vi "Pose3d_Log_Orig.vi"(9 "end Pose3d":T2={"Translation3d"={"X"=0.0, "Y"=0.0, "Z"=0.0}, "Rotation3d"={"Q_quaternion"={"R"=1.0, "V"=[0.0, 0.0, 0.0]}}} {"Translation3d"."Z" format="%14.3f"; "Translation3d"."Y" format="%14.3f"; "Translation3d"."X" format="%14.3f"}, 11 "in Pose3d":T2={"Translation3d"={"X"=0.0, "Y"=0.0, "Z"=0.0}, "Rotation3d"={"Q_quaternion"={"R"=1.0, "V"=[0.0, 0.0, 0.0]}}} {"Translation3d"."Z" format="%14.3f"; "Translation3d"."Y" format="%14.3f"; "Translation3d"."X" format="%14.3f"}) -> (3 "out Twist3d":T1)   [LabVIEW 2019]
doc: "Returns a Twist3d that maps this pose to the end pose. If c is the output of a.Log(b), then a.Exp(c) would yield b.\n \nParmeters:\n - IN POSE3D - The current POSE data structure\n - OTHER POSE3D - The end pose for the transformation.\n\nReturns:\n - OUT TWIST3D - The twist that maps this to end."
uses:
  FRC_LV_Trajectory_Library/Trajectory_Library.lvlib
  <vilib>/Analysis/Matrix/NI_Matrix.lvlib
  <vilib>/Analysis/Matrix/Numeric/Multiply/Multiply - RM,R.vi
  <vilib>/Analysis/Matrix/Numeric/Subtract/Subtract - RM,RM.vi
  <vilib>/Analysis/Matrix/Numeric/Add/Add - RM,RM.vi
  <vilib>/Analysis/NI_AALBase.lvlib
  <vilib>/Analysis/baseanly.llb/Real A x B.vi
  FRC_LV_Trajectory_Library/TypeDef/TWIST3D.ctl
  FRC_LV_Trajectory_Library/TypeDef/TRANSLATION3D.ctl
  FRC_LV_Trajectory_Library/TypeDef/QUATERNION.ctl
  FRC_LV_Trajectory_Library/TypeDef/ROTATION3D.ctl
  FRC_LV_Trajectory_Library/TypeDef/POSE3D.ctl
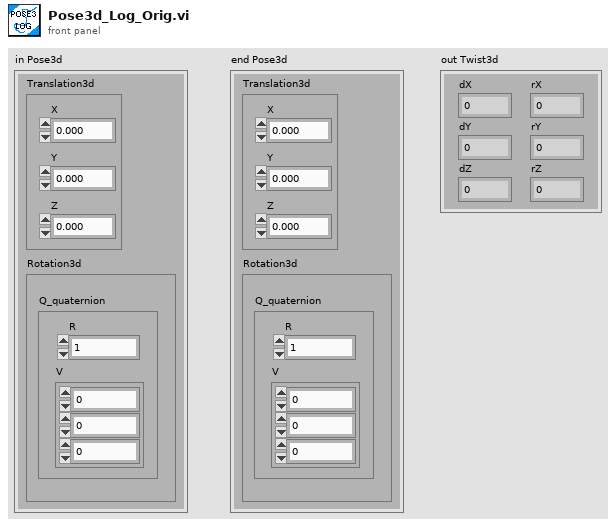
[diagram p1: front panel]
types:
  T1 = typedef "Trajectory_Library.lvlib/TWIST3D.ctl" = cluster{"dX":dbl, "dY":dbl, "dZ":dbl, "rX":dbl, "rY":dbl, "rZ":dbl}
  T2 = typedef "Trajectory_Library.lvlib/POSE3D.ctl" = cluster{"Translation3d":T3, "Rotation3d":T4}
  T3 = typedef "Trajectory_Library.lvlib/TRANSLATION3D.ctl" = cluster{"X":dbl, "Y":dbl, "Z":dbl}
  T4 = typedef "Trajectory_Library.lvlib/ROTATION3D.ctl" = cluster{"Q_quaternion":T5}
  T5 = typedef "Trajectory_Library.lvlib/QUATERNION.ctl" = cluster{"R":dbl, "V":dbl[]}
  T6 = typedef "NI_Matrix.lvlib/RealMatrix.ctl" = dbl[][]
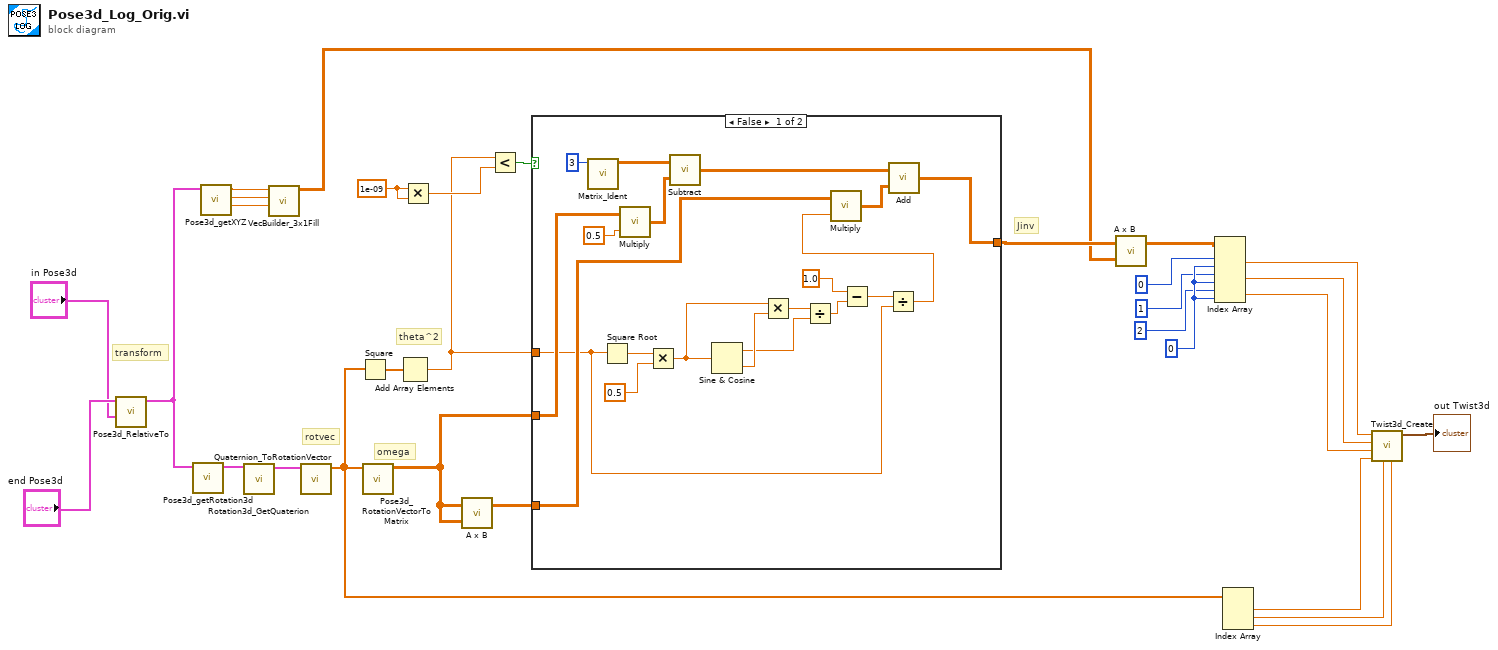
[diagram p0: block diagram]
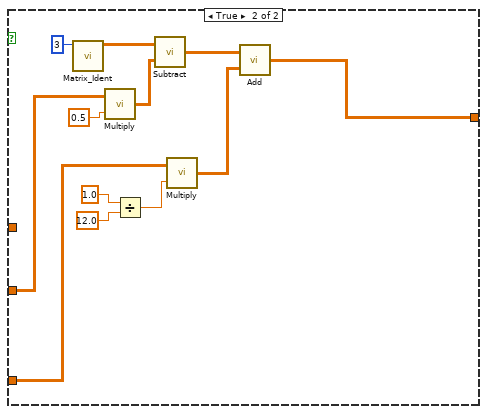
[diagram p2: hidden frame]
diagram:
  w7 = 0 ("index (col)")
  w20 = 1e-09 ("y")
  # "transform"
  # "Jinv"
  # "theta^2"
  # "rotvec"
  # "omega"
  n1 = call "Pose3d_RelativeTo.vi"("other Pose3d"="in Pose3d", "in Pose3d"="end Pose3d") -> ("out Pose3d"=w13:T2)  [unwired: 9 in]
  n2 = call "Pose3d_getRotation3d.vi"("in Pose3d"=w13) -> ("out Rotation3d"=w26:T4)  [unwired: 10 in]
  n3 = call "Pose3d_getXYZ.vi"("in Pose3d"=w13) -> ("Z"=w10:dbl, "Y"=w11:dbl, "X"=w12:dbl)  [unwired: 8 in]
  n4 = call "Rotation3d_GetQuaterion.vi"("in Rotation3d"=w26) -> ("out Quaterion"=w25:T5)  [unwired: 10 in]
  n5 = call "VecBuilder_3x1Fill.vi"("R2"=w10, "R1"=w11, "R0"=w12) -> ("output matrix"=w9:T6)  [unwired: 8 in]
  n6 = call "Quaternion_ToRotationVector.vi"("Quaternion"=w25) -> ("RotationVector"=w21:dbl[])  [unwired: 10 in]
  n7 = Square(x=w21) -> (x^2=w18:dbl[])
  n8 = call "Pose3d_RotationVectorToMatrix.vi"("RotationVector"=w21) -> ("Rotation Matrix"=w17:T6)  [unwired: 10 in]
  n9 = Add Array Elements(numeric array=w18) -> (sum=w15:dbl)
  n10 = Multiply(x=w20, y=w20) -> (x*y=w19:dbl)
  n11 = call-poly <vilib>:"A x B.vi"("B"=w17, "A"=w17) -> ("A x B"=w16:T6)  [unwired: 1 out]
  n12 = Less?(x=w15, y=w19) -> (x < y?=w28:bool)
  n13 = case shown="False" w28 {
    tunnel: w17 -> [w43 w60]
    tunnel: w16 -> [w40 w54]
    tunnel: [w31 w51] -> w14
    tunnel: w15 -> [w37 _]
    frame False {
      n14 = call "Matrix_Ident.vi"("Size"=3) -> ("output matrix"=w46:T6)  [unwired: 9 in, 1 out]
      n15 = Square Root(x=w37) -> (sqrt(x)=w50:dbl)
      n16 = call-poly <vilib>:"Multiply.vi"("Real Scalar c"=0.5 ("y"), "Real Matrix A"=w43) -> ("A * c"=w45:T6)
      n17 = Multiply(x=w50, y=0.5) -> (x*y=w39:dbl)
      n18 = call-poly <vilib>:"Subtract.vi"("Real Matrix B"=w45, "Real Matrix A"=w46) -> ("A - B"=w44:T6)
      n19 = Sine & Cosine(0:w39) -> (1:w35:dbl, 2:w38:dbl)
      n20 = Multiply(x=w39, y=w38) -> (x*y=w36:dbl)
      n21 = Divide(x=w36, y=w35) -> (x/y=w34:dbl)
      n22 = Subtract(x=1.0, y=w34) -> (x-y=w33:dbl)
      n23 = Divide(x=w33, y=w37) -> (x/y=w32:dbl)
      n24 = call-poly <vilib>:"Multiply.vi"("Real Scalar c"=w32, "Real Matrix A"=w40) -> ("A * c"=w41:T6)
      n25 = call-poly <vilib>:"Add.vi"("Real Matrix B"=w41, "Real Matrix A"=w44) -> ("A + B"=w31:T6)
    }
    frame True {
      n26 = call "Matrix_Ident.vi"("Size"=3) -> ("output matrix"=w59:T6)  [unwired: 9 in, 1 out]
      n27 = call-poly <vilib>:"Multiply.vi"("Real Scalar c"=0.5 ("y"), "Real Matrix A"=w60) -> ("A * c"=w58:T6)
      n28 = Divide(x=1.0, y=12.0) -> (x/y=w55:dbl)
      n29 = call-poly <vilib>:"Subtract.vi"("Real Matrix B"=w58, "Real Matrix A"=w59) -> ("A - B"=w53:T6)
      n30 = call-poly <vilib>:"Multiply.vi"("Real Scalar c"=w55, "Real Matrix A"=w54) -> ("A * c"=w52:T6)
      n31 = call-poly <vilib>:"Add.vi"("Real Matrix B"=w52, "Real Matrix A"=w53) -> ("A + B"=w51:T6)
    }
  }
  n32 = call-poly <vilib>:"A x B.vi"("B"=w9, "A"=w14) -> ("A x B"=w4:T6)  [unwired: 1 out]
  n33 = Index Array(array=w4, index (row) #1=0 ("index (row)"), index (col) #1=w7, index (row) #2=1 ("index (row)"), index (col) #2=w7, index (row) #3=2 ("index (row)"), index (col) #3=w7) -> (element #1=w3:dbl, element #2=w2:dbl, element #3=w1:dbl)
  n34 = Index Array(array=w21) -> (element #1=w22:dbl, element #2=w23:dbl, element #3=w24:dbl)  [unwired: 3 in]
  n35 = call "Twist3d_Create.vi"("rZ"=w24, "rY"=w23, "rX"=w22, "dZ"=w1, "dY"=w2, "dX"=w3) -> ("Twist3d"=→"out Twist3d":T1)  [unwired: 5 in]
